vi "Construct - Input.vi"(6 "Console Ref":refnum<vi>, 8 "Layout Type":refnum<class "Layout.lvclass">, 9 "Name":string, 10 "Level":T1=enum."DEBUG", 11 "buffer length":i32=1024) -> (0 "Error Out":errorcluster, 3 "Sink-Console":refnum<class "Sink-Console.lvclass">)   [LabVIEW 2019, in "TSC Event Logger.lvlib" / "Sink-Console.lvclass"]
uses:
  Sink-Console.lvclass
  C:/Development/Reuse-libraries/Event Logger/Log Sinks/Log Sinks.lvclass
  Log/Event Level.ctl
  Layouts/Layout.lvclass
  Layouts/SimpleLayout/SimpleLayout.lvclass
  C:/Development/Reuse-libraries/Event Logger/Layouts/Layout.lvclass
  Sink-Console.lvclass/Sink-Console.ctl
  Log Sinks.lvclass/Log Sinks.ctl
  Log Sinks.lvclass
  TSC Event Logger.lvlib
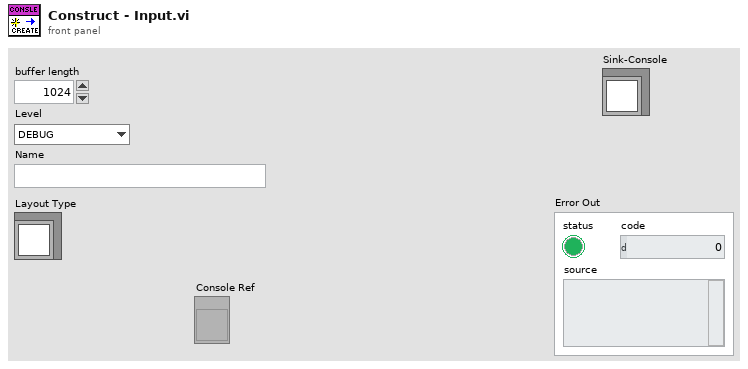
[diagram p1: front panel]
types:
  T1 = typedef "TSC Event Logger.lvlib/Event Level.ctl" = enum16{"OFF", "TRACE", "DEBUG", "INFO", "WARN", "ERROR", "FATAL"}
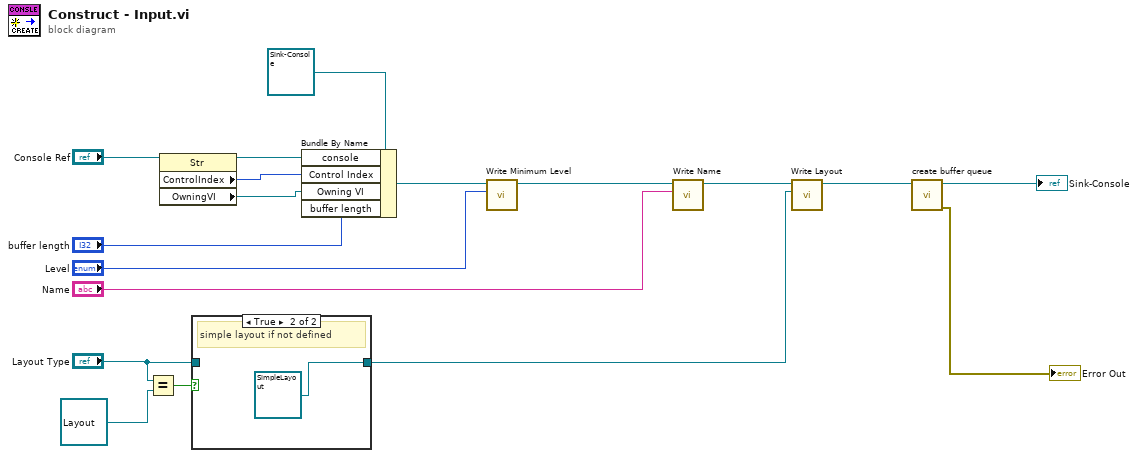
[diagram p0: block diagram]
diagram:
  n1 = Equal?(x="Layout Type", y=refnum<class "Layout.lvclass"> refnum ("TSC Event Logger.lvlib:Layout.lvclass")) -> (x = y?=w5:bool)
  n2 = property class="Str"(reference="Console Ref") -> (reference out=w14:refnum<vi>, "ControlIndex"=w15:i32, "OwningVI"=w16:refnum<vi>)  [unwired: 1 in, 1 out]
  n3 = case shown="True" w5 {
    tunnel: "Layout Type" -> [w19 _]
    tunnel: [w19 refnum<class "SimpleLayout.lvclass"> refnum ("TSC Event Logger.lvlib:SimpleLayout.lvclass")] -> w2
    frame False {
    }
    frame True {
      # "simple layout if not defined"
    }
  }
  n4 = Bundle By Name(cluster=refnum<class "Sink-Console.lvclass"> refnum ("TSC Event Logger.lvlib:Sink-Console.lvclass"), "console"=w14, "Control Index"=w15, "Owning VI"=w16, "buffer length"="buffer length") -> (w12:refnum<class "Sink-Console.lvclass">)
  n5 = call "Write Minimum Level.vi"("Level"="Level", "Log Sinks in"=w12) -> ("Log Sinks out"=w13:refnum<class "Sink-Console.lvclass">)  [unwired: 9 in]
  n6 = call "Write Name.vi"("Name"="Name", "Log Sinks in"=w13) -> ("Log Sinks out"=w11:refnum<class "Sink-Console.lvclass">)  [unwired: 9 in]
  n7 = call "Write Layout.vi"("Layout"=w2, "Log Sinks in"=w11) -> ("Log Sinks out"=w3:refnum<class "Sink-Console.lvclass">)  [unwired: 9 in]
  n8 = call "create buffer queue.vi"("Sink-Console in"=w3) -> ("error out"=→"Error Out":errorcluster, "Sink-Console out"=→"Sink-Console":refnum<class "Sink-Console.lvclass">)  [unwired: 9 in]
